vi "数字量输出统计结果.vi"   [LabVIEW 2010]
uses:
  全局量/自动测试结果.vi
  全局量/试验配置信息.vi
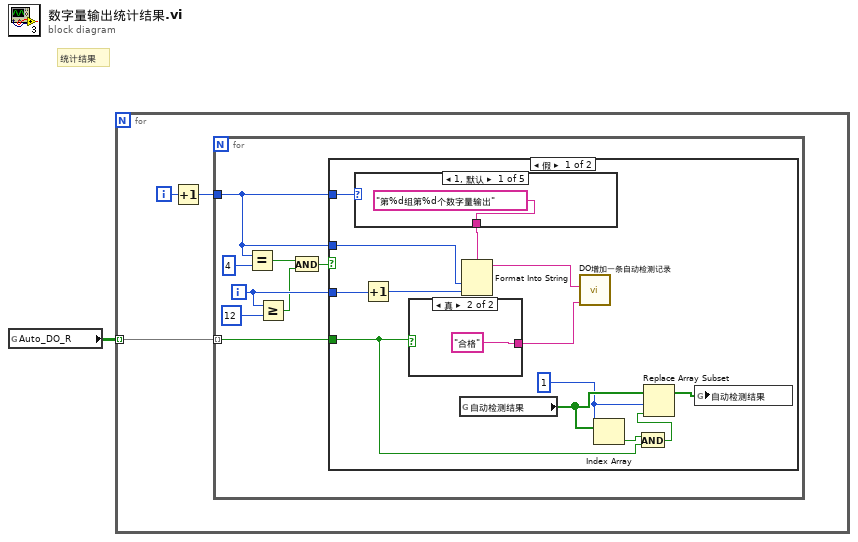
[diagram p0: block diagram]
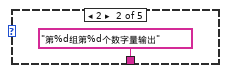
[diagram p2: hidden frame]
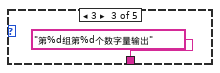
[diagram p3: hidden frame]
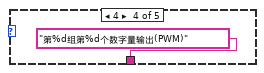
[diagram p4: hidden frame]
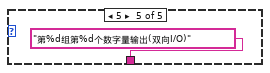
[diagram p5: hidden frame]
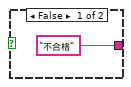
[diagram p6: hidden frame]
diagram:
  # "统计结果"
  n1 = global read "自动测试结果.vi" "Auto_DO_R"() -> (w1:bool[][])
  n2 = for {
    tunnel: w1 -> [w4] mode=indexing
    i -> [w3]
    n3 = Increment(x=w3) -> (x+1=w2:i32)
    n4 = for {
      tunnel: w4 -> [w12] mode=indexing
      tunnel: w2 -> [w5]
      i -> [w10]
      n5 = Equal?(x=w5, y=4) -> (x = y?=w8:bool)
      n6 = Greater Or Equal?(x=w10, y=12) -> (x >= y?=w7:bool)
      n7 = And(x=w8, y=w7) -> (x .and. y?=w6:bool)
      n8 = case shown="假" w6 {
        tunnel: w12 -> [w13 _]
        tunnel: w10 -> [w21 _]
        tunnel: w5 -> [w20 _]
        tunnel: w5 -> [w19 _]
        frame False {
          w16 = 1 ("索引")
          n9 = case shown="1, 默认" w19 {
            tunnel: ["第%d组第%d个数字量输出" "第%d组第%d个数字量输出" "第%d组第%d个数字量输出" "第%d组第%d个数字量输出(PWM)" "第%d组第%d个数字量输出(双向I/O)"] -> w25
            frame 1, Default {
            }
            frame 2 {
            }
            frame 3 {
            }
            frame 4 {
            }
            frame 5 {
            }
          }
          n10 = Increment(x=w21) -> (x+1=w24:i32)
          n11 = case shown="真" w13 {
            tunnel: ["不合格" "合格"] -> w22
            frame False {
            }
            frame True {
            }
          }
          n12 = global read "试验配置信息.vi" "自动检测结果"() -> (w17:bool[])
          n13 = Format Into String(format string=w25, w20, w24) -> (resulting string=w23:string)  [unwired: 2 in, 1 out]
          n14 = call "DO增加一条自动检测记录.vi"("测试结果"=w22, "测试内容"=w23) -> ()  [unwired: 10 in]
          n15 = Index Array(array=w17, index=w16) -> (element=w15:bool)
          n16 = And(x=w15, y=w13) -> (x .and. y?=w14:bool)
          n17 = Replace Array Subset(array=w17, new element=w14, index=w16) -> (w18:bool[])
          n18 = global write "试验配置信息.vi" "自动检测结果"(w18) -> ()
        }
        frame True {
        }
      }
    }
  }
